vi "Check_EnFlo_Tunnel_Cond.vi"() -> (0 "Status Cluster":T1, 1 "Heaters On?":bool)   [LabVIEW 2016]
uses:
  Anemometry/Anemometry Sub Vis/Gen Trav/Status_Cluster.ctl
  Anemometry/Anemometry Sub Vis/Gen Trav/Multi_Run_Status.ctl
  Anemometry/Anemometry Sub Vis/Controls/In_Range.ctl
  Anemometry/Anemometry Sub Vis/Globals/Meas_global.vi
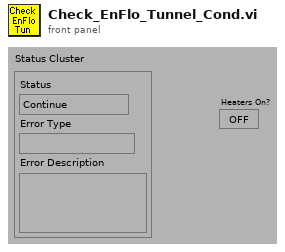
[diagram p1: front panel]
types:
  T1 = typedef "Status_Cluster.ctl" = cluster{"Status":T2, "Error Type":string, "Error Description":string}
  T2 = typedef "Multi_Run_Status.ctl" = enum16{"Continue", "Jump to Next Point", "Jump to Next Row", "Jump To Fall Back", "Terminate Run"}
  T3 = typedef "In_Range.ctl" = enum16{"%", "±", "% & ±"}
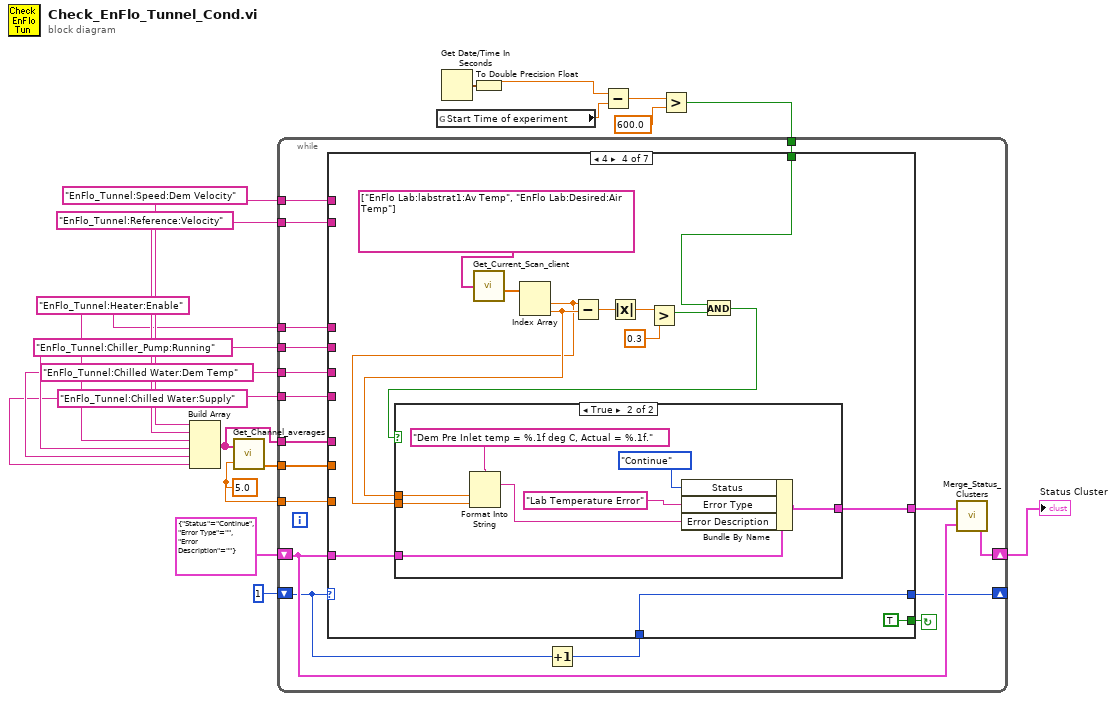
[diagram p0: block diagram]
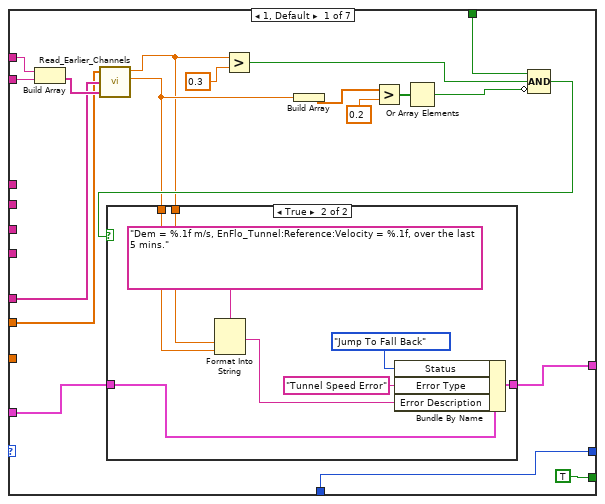
[diagram p2: hidden frame]
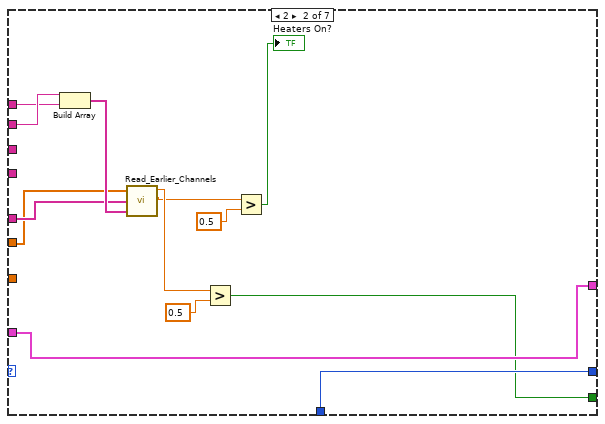
[diagram p4: hidden frame]
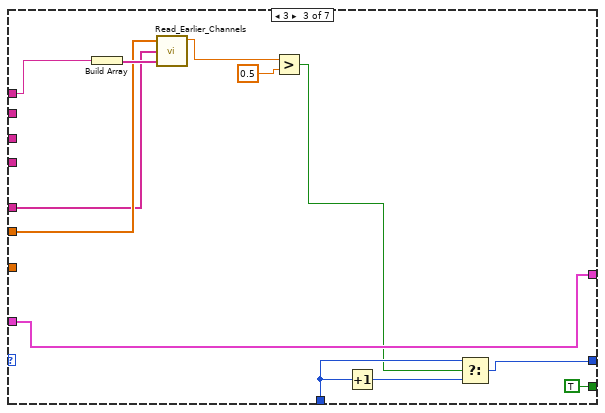
[diagram p5: hidden frame]
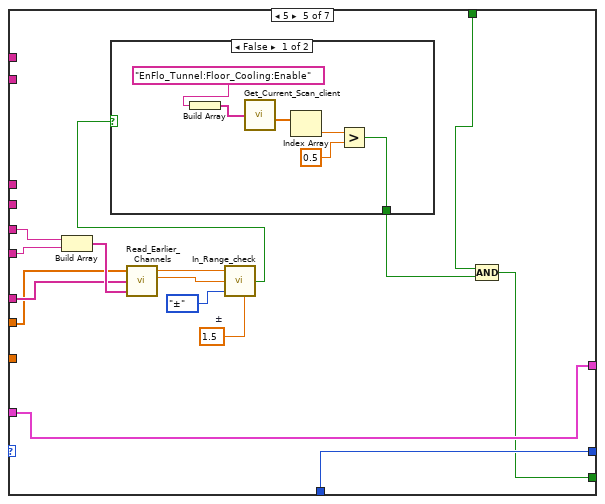
[diagram p7: hidden frame]
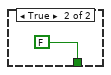
[diagram p8: hidden frame]
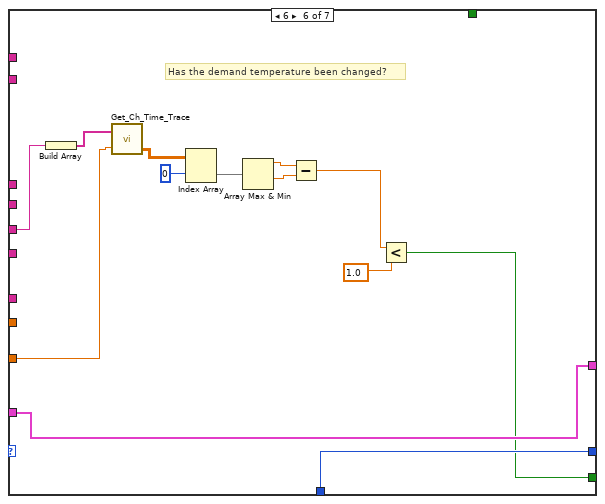
[diagram p9: hidden frame]
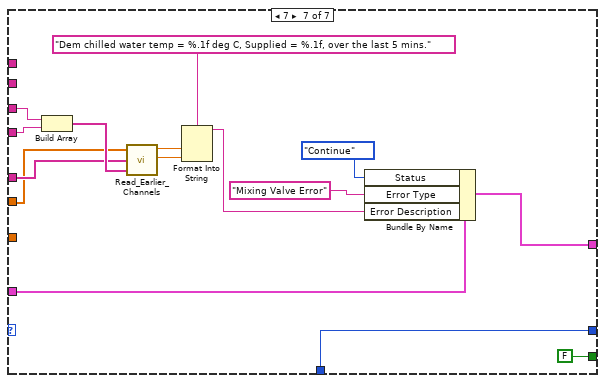
[diagram p10: hidden frame]
diagram:
  w8 = "EnFlo_Tunnel:Chilled Water:Supply"
  w9 = "EnFlo_Tunnel:Chilled Water:Dem Temp"
  w10 = "EnFlo_Tunnel:Chiller_Pump:Running"
  w15 = "EnFlo_Tunnel:Heater:Enable"
  w1 = 5.0 ("Averaging time (mins)")
  w17 = "EnFlo_Tunnel:Speed:Dem Velocity"
  w16 = "EnFlo_Tunnel:Reference:Velocity"
  n1 = Build Array(w17, w16, w15, w10, w9, w8) -> (w12:string[])
  n2 = call "Get_Channel_averages.vi"("Desired Ch Names"=w12, "Averaging time (mins)"=w1) -> ("number"=w18:dbl[])  [unwired: 1 in, 2 out]
  n3 = global read "Meas_global.vi" "Start Time of experiment"() -> (w5:dbl)
  n4 = Get Date/Time In Seconds() -> (seconds since 1Jan1904=w2:timestamp)
  n5 = To Double Precision Float(number=w2) -> (double precision float=w4:dbl)
  n6 = Subtract(x=w4, y=w5) -> (x-y=w6:dbl)
  n7 = Greater?(x=w6, y=600.0) -> (0:w3:bool)
  n8 = while {
    tunnel: w3 -> [w20]
    tunnel: w8 -> [w21]
    tunnel: w9 -> [w22]
    tunnel: w10 -> [w23]
    shift-left: 1 -> [w26]
    shift-right: [w25] -> _
    tunnel: w15 -> [w30]
    tunnel: w16 -> [w31]
    tunnel: w17 -> [w32]
    tunnel: w12 -> [w33]
    tunnel: w18 -> [w34]
    shift-left: T1 {"Status"=enum."Continue", "Error Type"="", "Error Description"=""} ("Status Cluster In") -> [w28]
    shift-right: [w27] -> w14
    tunnel: w1 -> [w19]
    stop <- w35 continue-if-true
    n9 = Increment(x=w26) -> (x+1=w24:i32)
    n10 = case shown="4" w26 {
      tunnel: [TRUE w69 TRUE TRUE w114 w142 FALSE] -> w35
      tunnel: w34 -> [w45 w73 w78 _ w123 _ w159]
      tunnel: w33 -> [w46 w74 w77 _ w124 _ w160]
      tunnel: w32 -> [w49 _ _ _ _ _ _]
      tunnel: w31 -> [w48 _ _ _ _ _ _]
      tunnel: w28 -> [w53 w76 w88 w96 w126 w146 w148]
      tunnel: [w51 w76 w88 w95 w126 w146 w147] -> w29
      tunnel: w30 -> [_ w67 w80 _ _ _ _]
      tunnel: w24 -> [w37 w72 w85 w92 w122 w145 w158]
      tunnel: [w37 w72 w86 w92 w122 w145 w158] -> w25
      tunnel: w23 -> [_ w71 _ _ _ _ _]
      tunnel: w22 -> [_ _ _ _ w121 w141 w156]
      tunnel: w21 -> [_ _ _ _ w120 _ w157]
      tunnel: w20 -> [w36 _ _ w90 w115 _ _]
      tunnel: w19 -> [_ _ _ _ _ w139 _]
      frame 1, Default {
        n11 = Build Array(w49, w48) -> (w47:string[])
        n12 = call "Read_Earlier_Channels.vi"("Present scan array"=w45, "Ch names"=w46, "Desired Channels"=w47) -> ("Index 0"=w43:dbl, "Index 1"=w44:dbl)  [unwired: 4 out]
        n13 = Greater?(x=w43, y=0.3) -> (0:w38:bool)
        n14 = Build Array(w44) -> (w41:dbl[])
        n15 = Greater?(x=w41, y=0.2) -> (0:w39:bool[])
        n16 = Or Array Elements(Boolean array=w39) -> (logical OR=w52:bool)
        n17 = Compound Arithmetic op=AND(w36, w38, invert w52) -> (w50:bool)
        n18 = case shown="True" w50 {
          tunnel: [w55 w62] -> w51
          tunnel: w53 -> [w55 w63]
          tunnel: w43 -> [_ w57]
          tunnel: w44 -> [_ w56]
          frame False {
          }
          frame True {
            n19 = Format Into String(format string="Dem = %.1f m/s, EnFlo_Tunnel:Reference:Velocity = %.1f, over the last 5 mins." ("Format String"), w57, w56) -> (resulting string=w58:string)  [unwired: 2 in, 1 out]
            n20 = Bundle By Name(cluster=w63, "Status"=Multi_Run_Status."Jump To Fall Back", "Error Type"="Tunnel Speed Error" ("Bundle Element"), "Error Description"=w58) -> (w62:T1)
          }
        }
      }
      frame 2 {
        n21 = Build Array(w71, w67) -> (w75:string[])
        n22 = call "Read_Earlier_Channels.vi"("Present scan array"=w73, "Ch names"=w74, "Desired Channels"=w75) -> ("Index 0"=w68:dbl, "Index 1"=w65:dbl)  [unwired: 4 out]
        n23 = Greater?(x=w68, y=0.5) -> (0:w69:bool)
        n24 = Greater?(x=w65, y=0.5) -> (0:→"Heaters On?":bool)
      }
      frame 3 {
        n25 = Build Array(w80) -> (w83:string[])
        n26 = call "Read_Earlier_Channels.vi"("Present scan array"=w78, "Ch names"=w77, "Desired Channels"=w83) -> ("Index 0"=w82:dbl)  [unwired: 5 out]
        n27 = Greater?(x=w82, y=0.5) -> (0:w79:bool)
        n28 = Increment(x=w85) -> (x+1=w84:i32)
        n29 = Select(t=w85, s=w79, f=w84) -> (s? t:f=w86:i32)
      }
      frame 4 {
        n30 = call "Get_Current_Scan_client.vi"("ADAM Ch Names"=string[] ["EnFlo Lab:labstrat1:Av Temp", "EnFlo Lab:Desired:Air Temp"] ("appended array")) -> ("Numerical Values"=w102:dbl[])  [unwired: 1 in, 2 out]
        n31 = Index Array(array=w102) -> (element #1=w93:dbl, element #2=w94:dbl)  [unwired: 2 in]
        n32 = Subtract(x=w93, y=w94) -> (x-y=w99:dbl)
        n33 = Absolute Value(x=w99) -> (abs(x)=w98:dbl)
        n34 = Greater?(x=w98, y=0.3 ("abs(x)")) -> (0:w91:bool)
        n35 = And(x=w90, y=w91) -> (x .and. y?=w89:bool)
        n36 = case shown="True" w89 {
          tunnel: w96 -> [w103 w108]
          tunnel: [w103 w107] -> w95
          tunnel: w94 -> [_ w106]
          tunnel: w93 -> [_ w105]
          frame False {
          }
          frame True {
            n37 = Format Into String(format string="Dem Pre Inlet temp = %.1f deg C, Actual = %.1f." ("Format String"), w106, w105) -> (resulting string=w109:string)  [unwired: 2 in, 1 out]
            n38 = Bundle By Name(cluster=w108, "Status"=Multi_Run_Status."Continue", "Error Type"="Lab Temperature Error" ("Bundle Element"), "Error Description"=w109) -> (w107:T1)
          }
        }
      }
      frame 5 {
        w117 = 1.5  # ±
        n39 = Build Array(w121, w120) -> (w125:string[])
        n40 = call "Read_Earlier_Channels.vi"("Present scan array"=w123, "Ch names"=w124, "Desired Channels"=w125) -> ("Index 0"=w119:dbl, "Index 1"=w118:dbl)  [unwired: 4 out]
        n41 = call "In_Range_check.vi"("±"=w117, "Mode"=In_Range."±", "Value"=w118, "Setpoint"=w119) -> ("In Range"=w113:bool)  [unwired: 1 in, 2 out]
        n42 = case shown="False" w113 {
          tunnel: [w127 FALSE] -> w112
          frame False {
            n43 = Build Array("EnFlo_Tunnel:Floor_Cooling:Enable") -> (w131:string[])
            n44 = call "Get_Current_Scan_client.vi"("ADAM Ch Names"=w131) -> ("Numerical Values"=w130:dbl[])  [unwired: 1 in, 2 out]
            n45 = Index Array(array=w130) -> (element=w129:dbl)  [unwired: 1 in]
            n46 = Greater?(x=w129, y=0.5) -> (0:w127:bool)
          }
          frame True {
          }
        }
        n47 = Compound Arithmetic op=AND(w115, w112) -> (w114:bool)
      }
      frame 6 {
        # "Has the demand temperature been changed?"
        n48 = Build Array(w141) -> (w140:string[])
        n49 = call "Get_Ch_Time_Trace.vi"("Desired Ch Names"=w140, "History Length (mins)"=w139) -> ("Output array"=w138:dbl[][])  [unwired: 2 out]
        n50 = Index Array(array=w138, index (row)=0 ("Index")) -> (element=w137:dbl[])  [unwired: 1 in]
        n51 = Array Max & Min(array=w137) -> (max value=w136:dbl, min value=w135:dbl)  [unwired: 2 out]
        n52 = Subtract(x=w136, y=w135) -> (x-y=w134:dbl)
        n53 = Less?(x=w134, y=1.0) -> (x < y?=w142:bool)
      }
      frame 7 {
        n54 = Build Array(w156, w157) -> (w161:string[])
        n55 = call "Read_Earlier_Channels.vi"("Present scan array"=w159, "Ch names"=w160, "Desired Channels"=w161) -> ("Index 0"=w150:dbl, "Index 1"=w149:dbl)  [unwired: 4 out]
        n56 = Format Into String(format string="Dem chilled water temp = %.1f deg C, Supplied = %.1f, over the last 5 mins." ("Format String"), w150, w149) -> (resulting string=w151:string)  [unwired: 2 in, 1 out]
        n57 = Bundle By Name(cluster=w148, "Status"=Multi_Run_Status."Continue", "Error Type"="Mixing Valve Error" ("Bundle Element"), "Error Description"=w151) -> (w147:T1)
      }
    }
    n58 = call "Merge_Status_Clusters.vi"("Status Cluster 2"=w28, "Status Cluster 1"=w29) -> ("Status Cluster Out"=w27:T1)
  }
  "Status Cluster" <- w14
